vi "graph to file.vi"(7 "file path (dialog if empty)":path, 8 "error in (no error)":errorcluster, 11 "Input array":cluster{cluster{dbl, "icn":dbl}[]}[](array[cluster])) -> (0 "error out":errorcluster)   [LabVIEW 2023]
uses:
  <vilib>/Utility/file.llb/Write Delimited Spreadsheet (DBL).vi
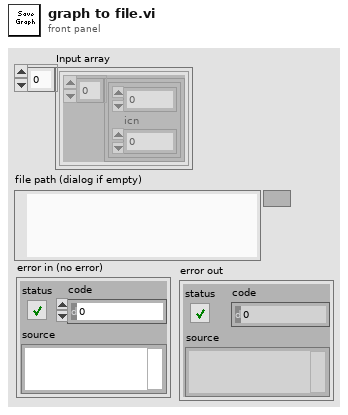
[diagram p1: front panel]
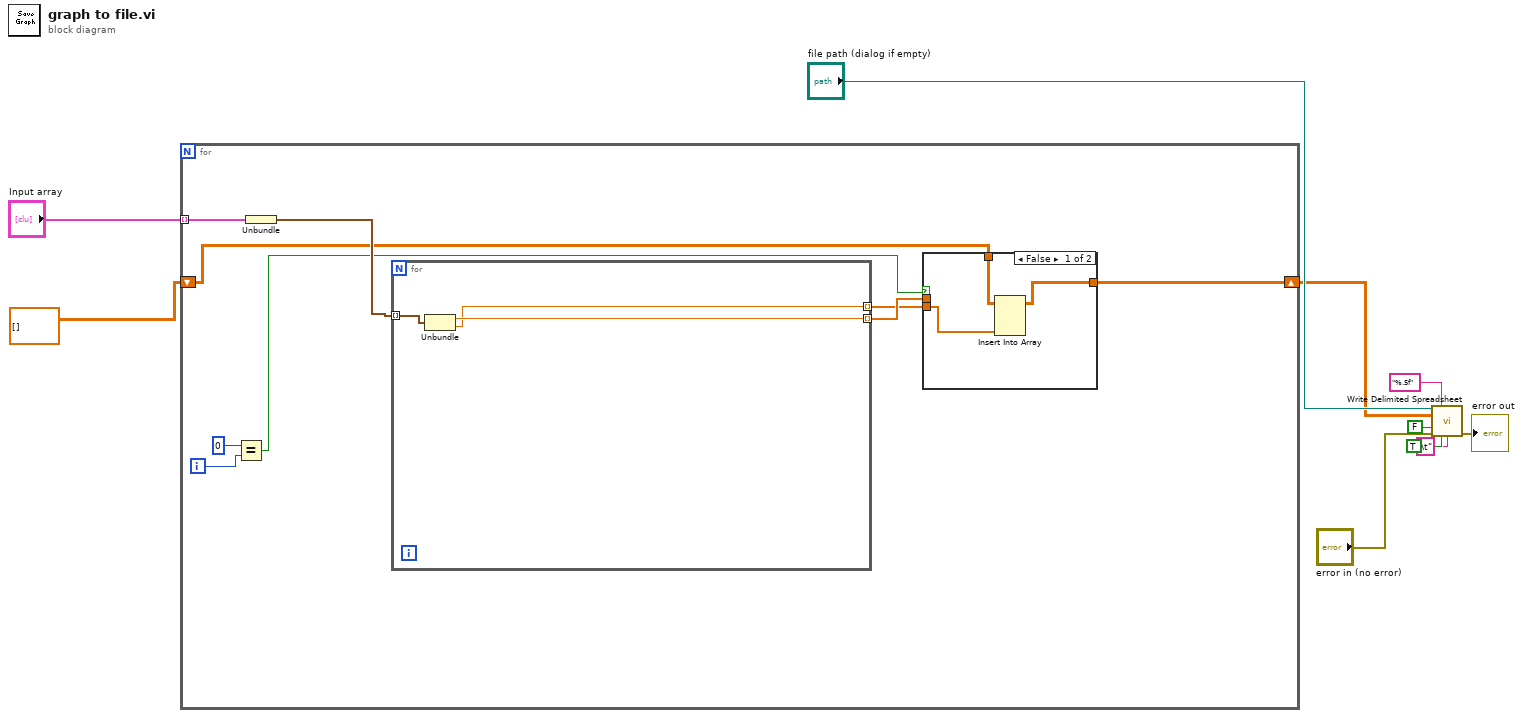
[diagram p0: block diagram]
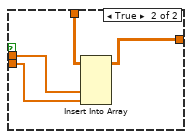
[diagram p2: hidden frame]
diagram:
  n1 = for {
    tunnel: "Input array" -> [w19] mode=indexing
    shift-right: [w11] -> w5
    shift-left: dbl[][] [] -> [w12]
    i -> [w18]
    n2 = Equal?(x=0, y=w18) -> (x = y?=w13:bool)
    n3 = Unbundle(w19) -> (w16:cluster{dbl, "icn":dbl}[])
    n4 = for {
      tunnel: w16 -> [w29] mode=indexing
      tunnel: [w28] -> w15 mode=indexing
      tunnel: [w27] -> w14 mode=indexing
      n5 = Unbundle(w29) -> (w28:dbl, "icn"=w27:dbl)
    }
    n6 = case shown="False" w13 {
      tunnel: w15 -> [_ w25]
      tunnel: w14 -> [w21 w24]
      tunnel: w12 -> [w22 w26]
      tunnel: [w20 w23] -> w11
      frame False {
        n7 = Insert Into Array(array=w22, new element=w21) -> (w20:dbl[][])  [unwired: 2 in]
      }
      frame True {
        n8 = Insert Into Array(array=w26, new element #1=w25, new element #2=w24) -> (w23:dbl[][])  [unwired: 2 in]
      }
    }
  }
  n9 = call-poly <vilib>:"Write Delimited Spreadsheet.vi"("file path (dialog if empty)"="file path (dialog if empty)", "format (%.3f)"="%.5f", "2D data"=w5, "append to file? (new file:F)"=FALSE, "error in (no error)"="error in (no error)", "transpose? (no:F)"=TRUE, "delimiter (\\t)"="\t" ("delimiter (\\t)")) -> ("error out"=→"error out":errorcluster)  [unwired: 7 in, 1 out]
